vi "Proxy Call Run.vi"(6 "Show Front-Panel":bool, 10 "API-Requests":T1, 11 "Actor in":refnum<class "Actor.lvclass">) -> (0 "error out":errorcluster, 3 "Actor out":refnum<class "Actor.lvclass">)   [LabVIEW 2018, in "Scripting.lvlib" / "Actor.lvlib" / "Interface.lvclass"]
uses:
  Interface.lvclass
  Actor.lvclass
  Actor/State.ctl
  Actor/Get State.ctl
  Actor/Stop.ctl
  Actor/Launch.ctl
  Actor/API-Requests.ctl
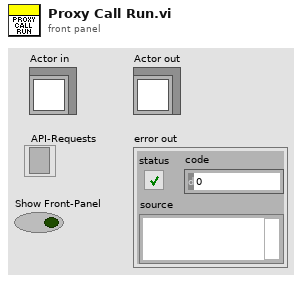
[diagram p1: front panel]
types:
  T1 = typedef "Scripting.lvlib/Actor.lvlib/Actor.lvclass/API-Requests.ctl" = refnum<event-registration>
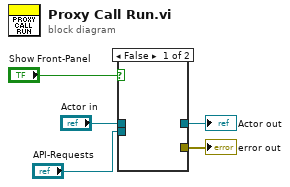
[diagram p0: block diagram]
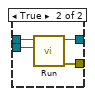
[diagram p2: hidden frame]
diagram:
  n1 = case shown="False" "Show Front-Panel" {
    tunnel: "API-Requests" -> [_ w9]
    tunnel: [_ w8] -> w4
    tunnel: [_ w7] -> w3
    tunnel: "Actor in" -> [_ w6]
    frame False {
    }
    frame True {
      n2 = call-dynamic "Run.vi"("API-Requests"=w9, "Actor in"=w6) -> ("error out"=w8:errorcluster, "Actor out"=w7:refnum<class "Actor.lvclass">)  [unwired: 8 in]
    }
  }
  "error out" <- w4
  "Actor out" <- w3
